vi "create tree item.vi"(7 "Item Type":T1=enum."Group", 8 "error in":errorcluster, 9 "found?":bool, 10 "Indent":i32, 11 "Left Cell String":string) -> (0 "error out":errorcluster, 3 "Item":T2)   [LabVIEW 2017]
uses:
  Tree Item Type.ctl
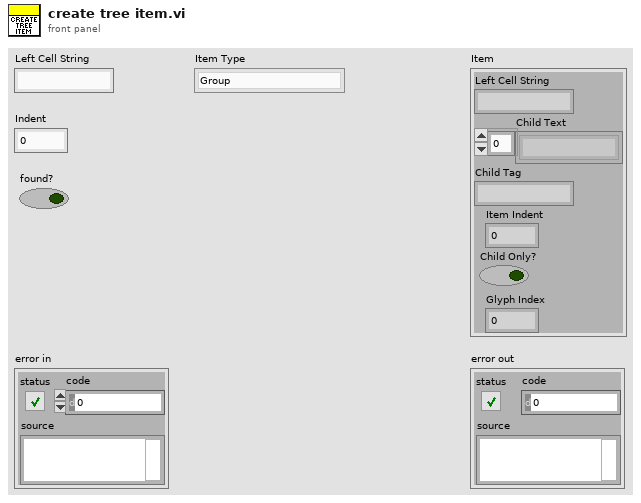
[diagram p1: front panel]
types:
  T1 = typedef "Tree Item Type.ctl" = enum16{"Plugin", "Group", "Transfer", "Channel", "Setting"}
  T2 = cluster{"Left Cell String":string, "Child Text":string[], "Child Tag":string, "Item Indent":i32, "Child Only?":bool, "Glyph Index":i32}
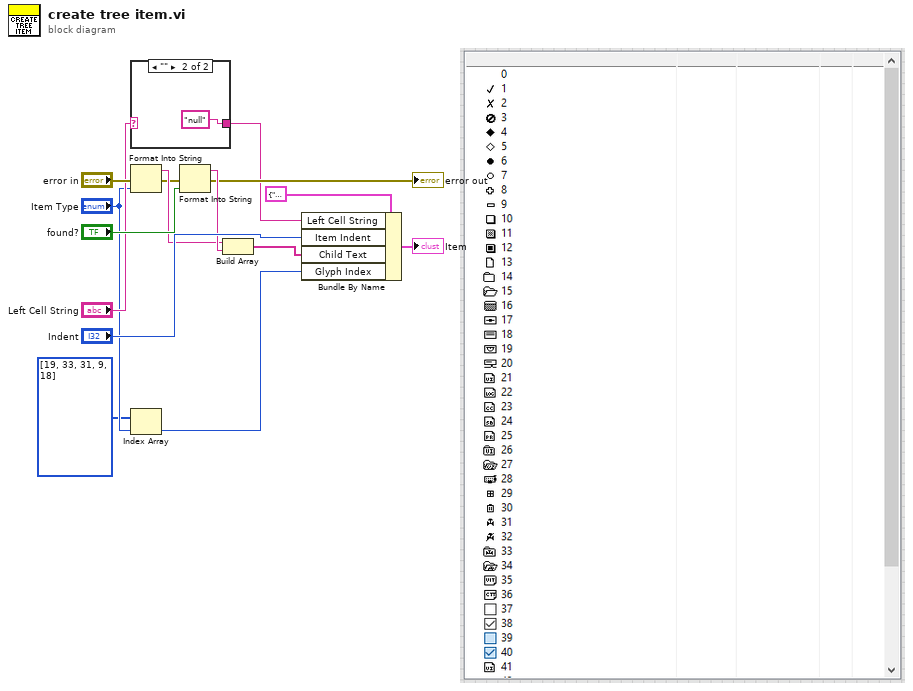
[diagram p0: block diagram]
diagram:
  n1 = case shown="\"\"" "Left Cell String" {
    selector: "Left Cell String" -> [w16 _]
    tunnel: [w16 "null"] -> w4
    frame Default {
    }
    frame "" {
    }
  }
  n2 = Format Into String(error in="error in", "Item Type") -> (resulting string=w9:string, error out=w7:errorcluster)  [unwired: 2 in]
  n3 = Index Array(array=i32[] [19, 33, 31, 9, 18] ("f"), index="Item Type") -> (element=w1:i32)
  n4 = Format Into String(error in=w7, "found?") -> (resulting string=w10:string, error out=→"error out":errorcluster)  [unwired: 2 in]
  n5 = Build Array(w9, w10) -> (w14:string[])
  n6 = Bundle By Name(cluster=T2 {"Left Cell String"="", "Child Text"=[], "Child Tag"="", "Item Indent"=0, "Child Only?"=FALSE, "Glyph Index"=0} ("Item"), "Left Cell String"=w4, "Item Indent"="Indent", "Child Text"=w14, "Glyph Index"=w1) -> (→"Item":T2)
